vi "Dissconnect.vi"(8 "error in (no error)":errorcluster, 11 "TCP_serverGUI in":refnum<class "TCP_serverGUI.lvclass">) -> (0 "error out":errorcluster, 3 "TCP_serverGUI out":refnum<class "TCP_serverGUI.lvclass">)   [LabVIEW 2023, in "TCP_serverGUI.lvlib" / "TCP_serverGUI.lvclass"]
uses:
  TCP_serverGUI.lvclass
  C:/Program Files (x86)/National Instruments/LabVIEW 2023/vi.lib/ActorFramework/Actor/Actor.lvclass
  <vilib>/ActorFramework/Actor/Actor.lvclass/Actor.ctl
  TCP_serverGUI.lvclass/TCP_serverGUI.ctl
  TCP_ServerWithGUI Messages/CloseConnection Msg/CloseConnection Msg.lvclass/CloseConnection Msg.ctl
  <vilib>/ActorFramework/Message Enqueuer/Message Enqueuer.lvclass/Message Enqueuer.ctl
  <vilib>/ActorFramework/Message Enqueuer/Enqueue.vi
  TCP_ServerWithGUI Messages/CloseConnection Msg/CloseConnection Msg.lvclass
  C:/Program Files (x86)/National Instruments/LabVIEW 2023/vi.lib/ActorFramework/Message/Message.lvclass
  <vilib>/ActorFramework/Message Priority Queue/Priority Enqueue.vi
  <vilib>/ActorFramework/Actor/Actor.lvclass
  C:/Source/LabVIEW/TCP_server/TCP_serverGUI/TCP_serverGUI/TCP_serverGUI.lvclass
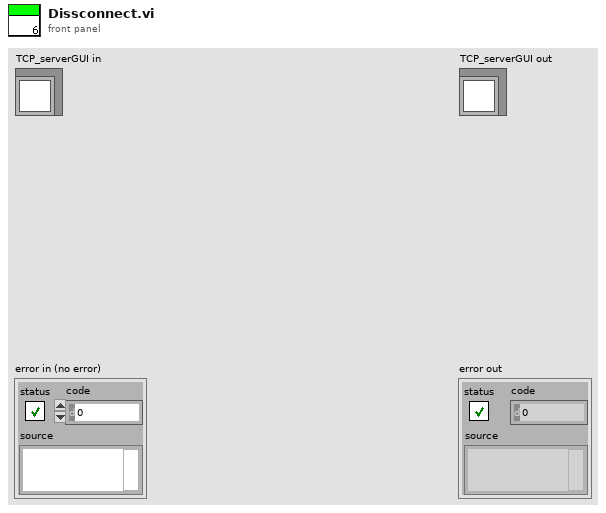
[diagram p1: front panel]
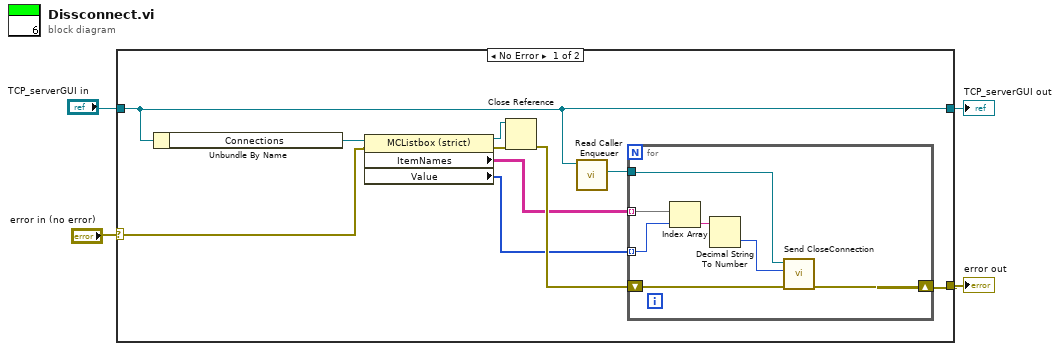
[diagram p0: block diagram]
diagram:
  n1 = case shown="No Error" "error in (no error)" {
    selector: "error in (no error)" -> [w11 w23]
    tunnel: [w7 w23] -> w3
    tunnel: [w10 w22] -> w1
    tunnel: "TCP_serverGUI in" -> [w10 w22]
    frame No Error {
      n2 = Unbundle By Name(w10) -> ("Connections"=w14:refnum<vi>)
      n3 = property class="MCListbox (strict)"(reference=w14, error in=w11) -> (reference out=w12:refnum<vi>, error out=w13:errorcluster, "ItemNames"=w5:string[][], "Value"=w6:i32[])
      n4 = Close Reference(reference=w12, error in (no error)=w13) -> (error out=w8:errorcluster)
      n5 = call <vilib>:"Read Caller Enqueuer.vi"("Actor"=w10) -> ("Caller Enqueuer"=w9:refnum<class "Message Enqueuer.lvclass">)  [unwired: 10 in]
      n6 = for {
        tunnel: w6 -> [w17] mode=indexing
        tunnel: w9 -> [w21]
        shift-right: [w19] -> w7
        shift-left: w8 -> [w20]
        tunnel: w5 -> [w18] mode=indexing
        n7 = Index Array(array=w18, index=w17) -> (element=w16:string)
        n8 = Decimal String To Number(string=w16) -> (number=w15:i32)  [unwired: 2 in, 1 out]
        n9 = call "Send CloseConnection.vi"("error in (no error)"=w20, "Connection Number"=w15, "Message Enqueuer"=w21) -> ("error out"=w19:errorcluster)  [unwired: 7 in, 1 out]
      }
    }
    frame Error {
    }
  }
  "error out" <- w3
  "TCP_serverGUI out" <- w1
